vi "For Loop.vi"() -> ()   [LabVIEW 2021]
panel:
  out "Factorial":i32
  in  "Numeric":i32
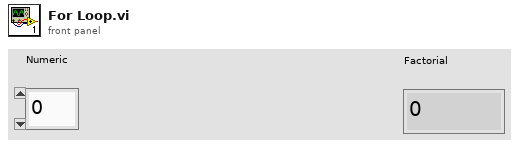
[diagram p1: front panel]
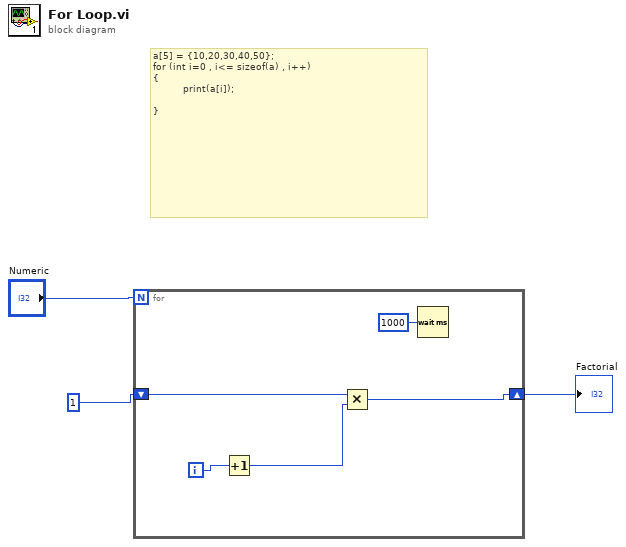
[diagram p0: block diagram]
diagram:
  # "a[5] = {10,20,30,40,50};\nfor (int i=0 , i<= sizeof(a) , i++)\n{\n          print(a[i]);\n\n}"
  n1 = for {
    N: "Numeric" -> [_]
    shift-right: [w7] -> w1
    shift-left: 1 -> [w8]
    i -> [w6]
    n2 = Increment(x=w6) -> (x+1=w5:i32)
    n3 = Multiply(x=w8, y=w5) -> (x*y=w7:i32)
    n4 = Wait (ms)(milliseconds to wait=u32 1000) -> ()  [unwired: 1 out]
  }
  "Factorial" <- w1
